vi "IsNullReferenceCheck.vi"(7 "error in":errorcluster, 8 "MCanHandleIn":T1) -> (2 "error out":errorcluster, 3 "MCanHandleOut":T1)   [LabVIEW 2011, in "Konvolucio MCAN120803.lvlib"]
uses:
  <instrlib>/Konvolucio MCAN120803/Konvolucio MCAN120803.lvlib
  <instrlib>/Konvolucio MCAN120803/Types/CanHandleType.ctl
  C:/Program Files/National Instruments/LabVIEW 2011/instr.lib/Konvolucio MCAN120803/Private/Konvolucio.MCAN120803.API.dll
  Konvolucio.MCAN120803.API.dll
panel:
  out "call chain":string[](array[string])
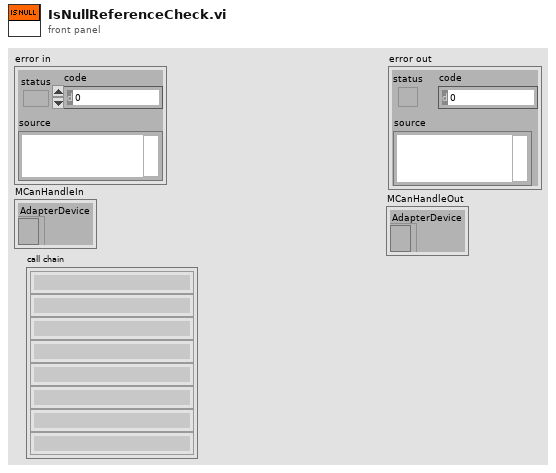
[diagram p1: front panel]
types:
  T1 = typedef "Konvolucio MCAN120803.lvlib/CanHandleType.ctl" = cluster{"AdapterDevice":refnum<k24>}
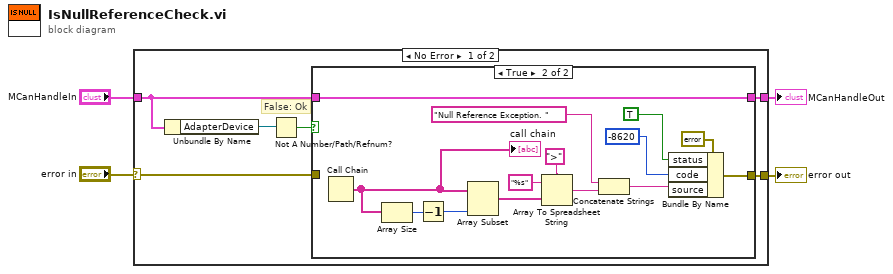
[diagram p0: block diagram]
diagram:
  n1 = case shown="No Error" "error in" {
    selector: "error in" -> [w5 w27]
    tunnel: [w9 w27] -> w4
    tunnel: [w8 w28] -> w3
    tunnel: "MCanHandleIn" -> [w7 w28]
    frame No Error {
      # "False: Ok"
      n2 = Unbundle By Name(w7) -> ("AdapterDevice"=w10:refnum<k24>)
      n3 = Not A Number/Path/Refnum?(number/path/refnum=w10) -> (NaN/Path/Refnum?=w6:bool)
      n4 = case shown="True" w6 {
        tunnel: [w11 w18] -> w9
        tunnel: [w12 w26] -> w8
        tunnel: w7 -> [w12 w26]
        tunnel: w5 -> [w11 _]
        frame False {
        }
        frame True {
          n5 = Call Chain() -> (call chain=w23:string[])
          "call chain" <- w23
          n6 = Array Size(array=w23) -> (size(s)=w24:i32)
          n7 = Decrement(x=w24) -> (x-1=w25:i32)
          n8 = Array Subset(array=w23, length=w25) -> (w22:string[])  [unwired: 1 in]
          n9 = Array To Spreadsheet String(delimiter (Tab)=">", array=w22, 3:"%s" ("format string")) -> (spreadsheet string=w15:string)
          n10 = Concatenate Strings("Null Reference Exception. " ("source"), w15) -> (w13:string)
          n11 = Bundle By Name(cluster=errorcluster {"status"=FALSE, "code"=0, "source"=""} ("input cluster"), "status"=TRUE, "code"=-8620, "source"=w13) -> (w18:errorcluster)
        }
      }
    }
    frame Error {
    }
  }
  "error out" <- w4
  "MCanHandleOut" <- w3
